vi "initialise.vi"(8 "error in (no error)":errorcluster, 11 "CQT_DDS in":refnum<class "CQT_DDS.lvclass">) -> (0 "error out":errorcluster, 3 "CQT_DDS out":refnum<class "CQT_DDS.lvclass">)   [LabVIEW 2009, in "Hardware.lvlib" / "Channels.lvlib" / "CQT_DDS.lvclass"]
uses:
  CQT_DDS.lvclass
  CQT_DDS.lvclass/CQT_DDS.ctl
  C:/Program Files/National Instruments/LabVIEW 2009/instr.lib/CQT_DDS/DDSLibrary/20111109/CQTAD9958.dll
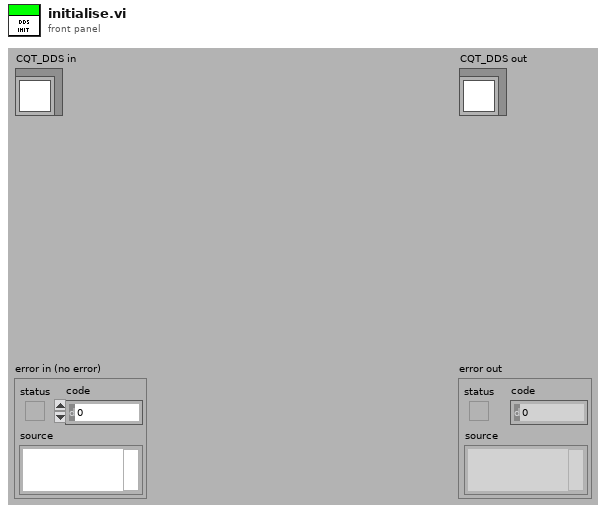
[diagram p1: front panel]
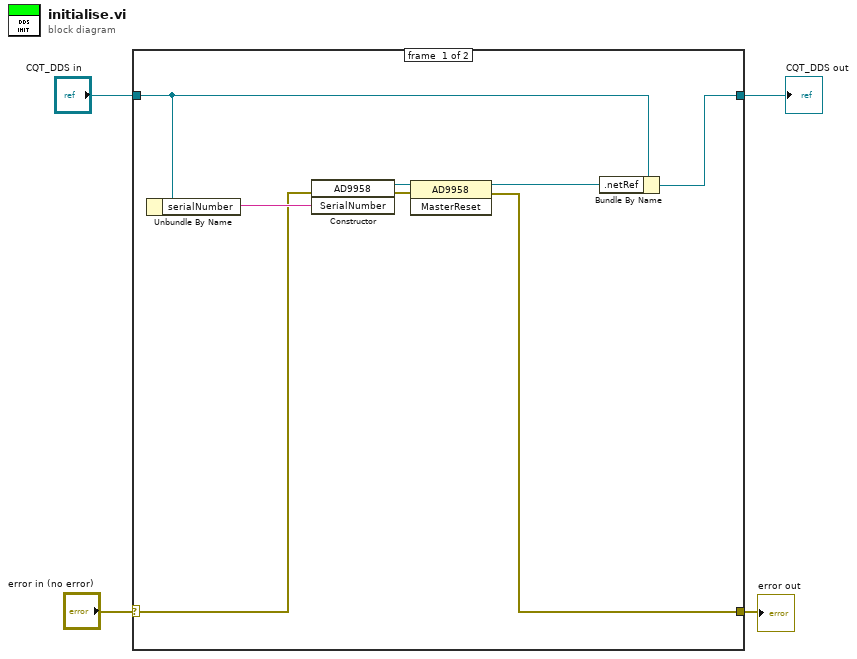
[diagram p0: block diagram]
diagram:
  n1 = case shown="No Error" "error in (no error)" {
    selector: "error in (no error)" -> [w6 w13]
    tunnel: [w9 w13] -> w3
    tunnel: [w10 w14] -> w2
    tunnel: "CQT_DDS in" -> [w11 w14]
    frame #0 {
      n2 = Unbundle By Name(w11) -> ("serialNumber"=w7:string)
      n3 = constructor class="AD9958"(error in=w6, "SerialNumber"=w7) -> (reference out=w5:refnum<k24>, error out=w8:errorcluster)  [unwired: 2 in, 2 out]
      n4 = invoke class="AD9958" method="MasterReset"(reference=w5, error in=w8) -> (reference out=w12:refnum<k24>, error out=w9:errorcluster)  [unwired: 1 in, 1 out]
      n5 = Bundle By Name(cluster=w11, ".netRef"=w12) -> (w10:refnum<class "CQT_DDS.lvclass">)
    }
    frame #1 {
    }
  }
  "error out" <- w3
  "CQT_DDS out" <- w2
